vi "UDP - Write CMD.vi"(6 "V2":bool, 7 "CMD":T6, 8 "error in":errorcluster, 10 "Data":T5={"Test"={"Target Load"=0.0, "Target Disp"=0.0, "Rate"=0.0, "Speed"=0.0}, "Sensor"={"Name"=[], "Unit"=[], "Decimal Point"=[], "Ch Log"=[], "H Alarm"=[], "L Alarm"=[], "H Limit"=[], "L Limit"=[], "Filter"=[], "Gain"=[], "Calib Type"=[]}, "PID"={"SP"=-2.7823365e-08, "PV"=-3.023652e-13, "kP"=8.5432666e-24, "kI"=2.29252e-41, "kD"=1.570387e-38, "FF"=25.0, "Err Band"=0.0, "Max"=15, "Min"=-7, "Ts"=1886611780, "Out"=0, "Mode"=0}, "ADC"={"Active Ch"=[255, 255, 255, 0, 0, 0, 0, 0], "Filter Type"=2, "Post Filter"=[1, 1, 1, 1, 0, 200, 66, 184], "Gain"=[0, 0, 0, 0, 0, 122, 68, 0], "FS"=32, "IntOC"=0, "IntFC"=255, "SysOC"=255, "Cofficient"=[1.0, 1.0, 1.0, 1.0, 1.0, 1.0, 1.0, 1.0], "K"=[1.2450000047683716, 1.2450000047683716], "Max"=1048576}, "System"={"Out Type"=0, "Inverse"=0, "Monitor"=0, "Reserve"=0, "ACC Time"=0, "Pulse Rev"=0, "Stroke"=0, "Auto Off"=0, "Gear Ratio"=0.0, "Pitch"=0.0, "Max Speed"=0, "Jog Speed"=0, "Disp Coff"=0.0, "Max Load"=0}, "Index"=enum."Ch1", "Datalog"=enum."Empty"}, 11 "UDP Info":T7) -> (0 "error out":errorcluster, 1 "IP Address":string, 2 "Data Out":T4 {"Status" items=["Stop", "Ramp Up", "Ramp Down", "Jog Up", "Jog Down", "PID Mode", "PID Ramp"]; "Event" items=["Stop", "Running", "PID", "Up Limit", "Down Limit", "Load Limit"]}, 3 "UDP Info Out":T7, 4 "Success":bool, 5 "data out":string, 9 "Channels 2":T1)   [LabVIEW 2019]
uses:
  Controls/UDP - Command.ctl
  Controls/Communication - Write Data.ctl
  Controls/UDP - Status.ctl
  Controls/UDP - Event.ctl
  Controls/Global - Data UDP.vi
panel:
  out "x+y":i32
  out "appended array":u8[](array[numeric])
  out "CMD":string
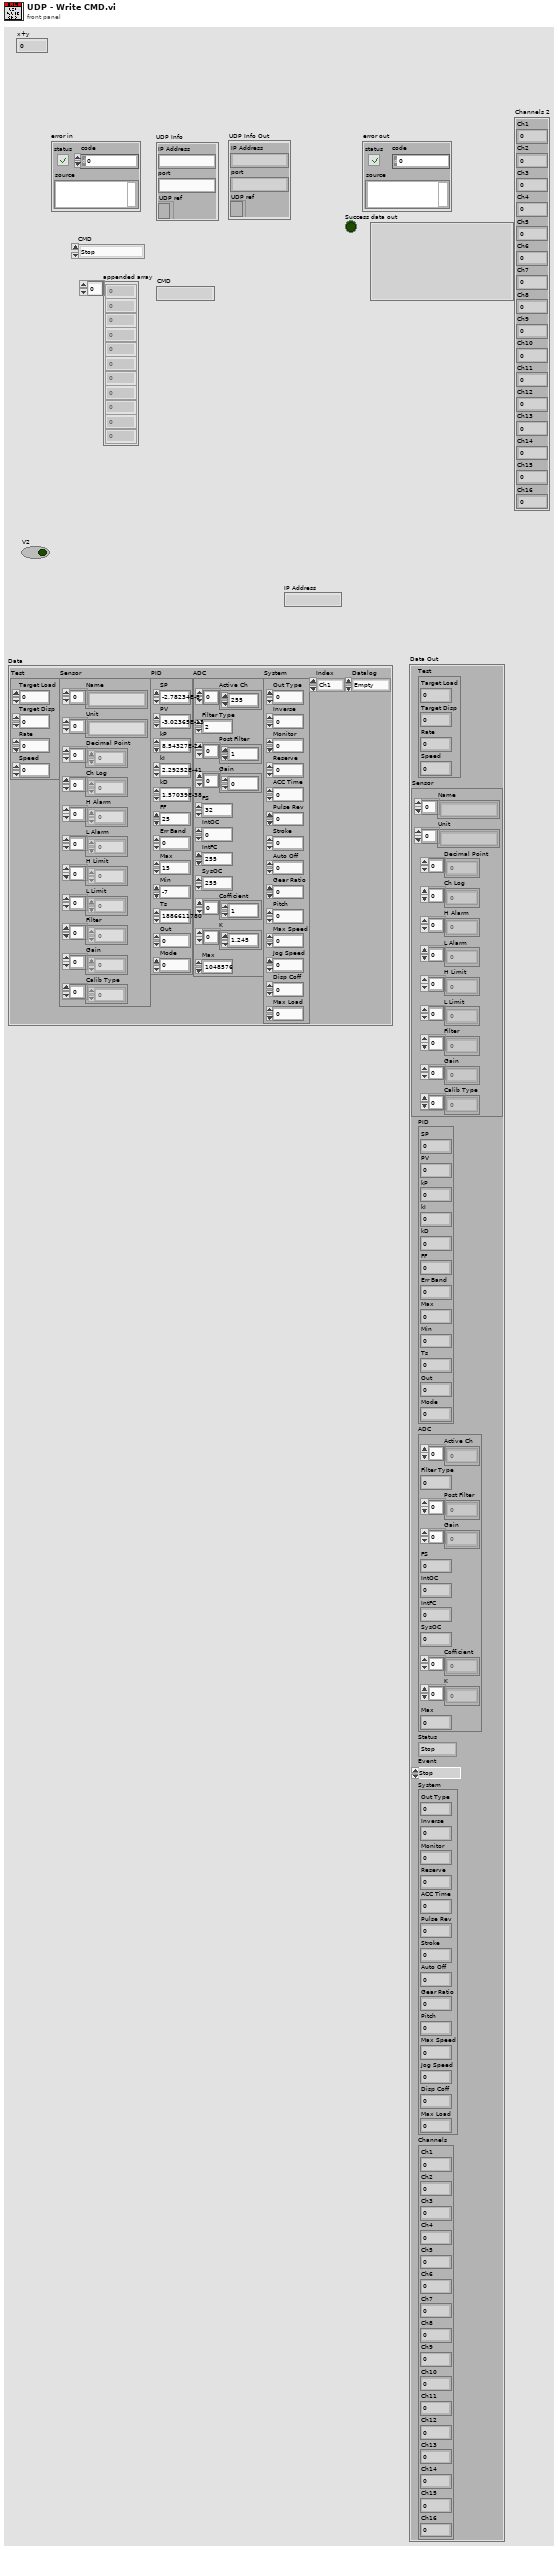
[diagram p1: front panel]
types:
  T1 = cluster{"Ch1":sgl, "Ch2":sgl, "Ch3":sgl, "Ch4":sgl, "Ch5":sgl, "Ch6":sgl, "Ch7":sgl, "Ch8":sgl, "Ch9":sgl, "Ch10":sgl, "Ch11":sgl, "Ch12":sgl, "Ch13":sgl, "Ch14":sgl, "Ch15":sgl, "Ch16":sgl}
  T2 = typedef "UDP - Status.ctl" = u16
  T3 = typedef "UDP - Event.ctl" = u16
  T4 = cluster{"Test":cluster{"Target Load":sgl, "Target Disp":sgl, "Rate":sgl, "Speed":sgl}, "Sensor":cluster{"Name":string[], "Unit":string[], "Decimal Point":u8[], "Ch Log":u8[], "H Alarm":u8[], "L Alarm":u8[], "H Limit":sgl[], "L Limit":sgl[], "Filter":u8[], "Gain":u8[], "Calib Type":u32[]}, "PID":cluster{"SP":sgl, "PV":sgl, "kP":sgl, "kI":sgl, "kD":sgl, "FF":sgl, "Err Band":sgl, "Max":i32, "Min":i32, "Ts":u32, "Out":i32, "Mode":u8}, "ADC":cluster{"Active Ch":u8[], "Filter Type":u8, "Post Filter":u8[], "Gain":u8[], "FS":u16, "IntOC":u8, "IntFC":u8, "SysOC":u8, "Cofficient":dbl[], "K":dbl[], "Max":i32}, "Status":T2, "Event":T3, "System":cluster{"Out Type":u8, "Inverse":u8, "Monitor":u8, "Reserve":u8, "ACC Time":u32, "Pulse Rev":u32, "Stroke":u32, "Auto Off":u32, "Gear Ratio":sgl, "Pitch":sgl, "Max Speed":u32, "Jog Speed":u32, "Disp Coff":sgl, "Max Load":u32}, "Channels":cluster{"Ch1":sgl, "Ch2":sgl, "Ch3":sgl, "Ch4":sgl, "Ch5":sgl, "Ch6":sgl, "Ch7":sgl, "Ch8":sgl, "Ch9":sgl, "Ch10":sgl, "Ch11":sgl, "Ch12":sgl, "Ch13":sgl, "Ch14":sgl, "Ch15":sgl, "Ch16":sgl}}
  T5 = typedef "Communication - Write Data.ctl" = cluster{"Test":cluster{"Target Load":sgl, "Target Disp":sgl, "Rate":sgl, "Speed":sgl}, "Sensor":cluster{"Name":string[], "Unit":string[], "Decimal Point":u8[], "Ch Log":u8[], "H Alarm":u8[], "L Alarm":u8[], "H Limit":sgl[], "L Limit":sgl[], "Filter":u8[], "Gain":u8[], "Calib Type":u32[]}, "PID":cluster{"SP":sgl, "PV":sgl, "kP":sgl, "kI":sgl, "kD":sgl, "FF":sgl, "Err Band":sgl, "Max":i32, "Min":i32, "Ts":u32, "Out":i32, "Mode":u8}, "ADC":cluster{"Active Ch":u8[], "Filter Type":u8, "Post Filter":u8[], "Gain":u8[], "FS":u16, "IntOC":u8, "IntFC":u8, "SysOC":u8, "Cofficient":dbl[], "K":dbl[], "Max":i32}, "System":cluster{"Out Type":u8, "Inverse":u8, "Monitor":u8, "Reserve":u8, "ACC Time":u32, "Pulse Rev":u32, "Stroke":u32, "Auto Off":u32, "Gear Ratio":sgl, "Pitch":sgl, "Max Speed":u32, "Jog Speed":u32, "Disp Coff":sgl, "Max Load":u32}, "Index":enum16{"Ch1", "Ch2", "Ch3", "Ch4", "Ch5", "Ch6", "Ch7", "Ch8", "Ch9", "Ch10", "Ch11", "Ch12", "Ch13", "Ch14", "Ch15", "Ch16"}, "Datalog":enum16{"Ch1-Ch16", "Ch17-Ch32", "Ch32-Ch48", "Ch49-Ch64", "Empty"}}
  T6 = typedef "UDP - Command.ctl" = enum16{"Stop", "Jog Up", "Jog Down", "Ramp Up", "Ramp Down", "PID Target", "PID Ramp", "Disp Run", "Read Ch Data", "Zero Channel", "Zero Disp", "Read Sensor", "Write Sensor", "Read ADC", "Write ADC", "Read PID", "Write PID", "Read Test", "Write Test", "Read System", "Write System", "Read Datalog", "Read Datalog Sensor"}
  T7 = cluster{"IP Address":string, "port":string, "UDP ref":refnum<k16>}
  T8 = cluster{"Out Type":u8, "Inverse":u8, "Monitor":u8, "Reserve":u8, "ACC Time":u32, "Pulse Rev":u32, "Stroke":u32, "Auto Off":u32, "Gear Ratio":sgl, "Pitch":sgl, "Max Speed":u32, "Jog Speed":u32, "Disp Coff":sgl, "Max Load":u32}
  T9 = cluster{"Name":string[], "Unit":string[], "Decimal Point":u8[], "Ch Log":u8[], "H Alarm":u8[], "L Alarm":u8[], "H Limit":sgl[], "L Limit":sgl[], "Filter":u8[], "Gain":u8[], "Calib Type":u32[]}
  T10 = cluster{"Active Ch":u8[], "Filter Type":u8, "Post Filter":u8[], "Gain":u8[], "FS":u16, "IntOC":u8, "IntFC":u8, "SysOC":u8, "Cofficient":dbl[], "K":dbl[], "Max":i32}
  T11 = cluster{"Target Load":sgl, "Target Disp":sgl, "Rate":sgl, "Speed":sgl}
  T12 = cluster{"SP":sgl, "PV":sgl, "kP":sgl, "kI":sgl, "kD":sgl, "FF":sgl, "Err Band":sgl, "Max":i32, "Min":i32, "Ts":u32, "Out":i32, "Mode":u8}
  T13 = cluster{"Target Load":sgl, "Target Disp":sgl, "Rate":sgl, "Ch4":sgl}
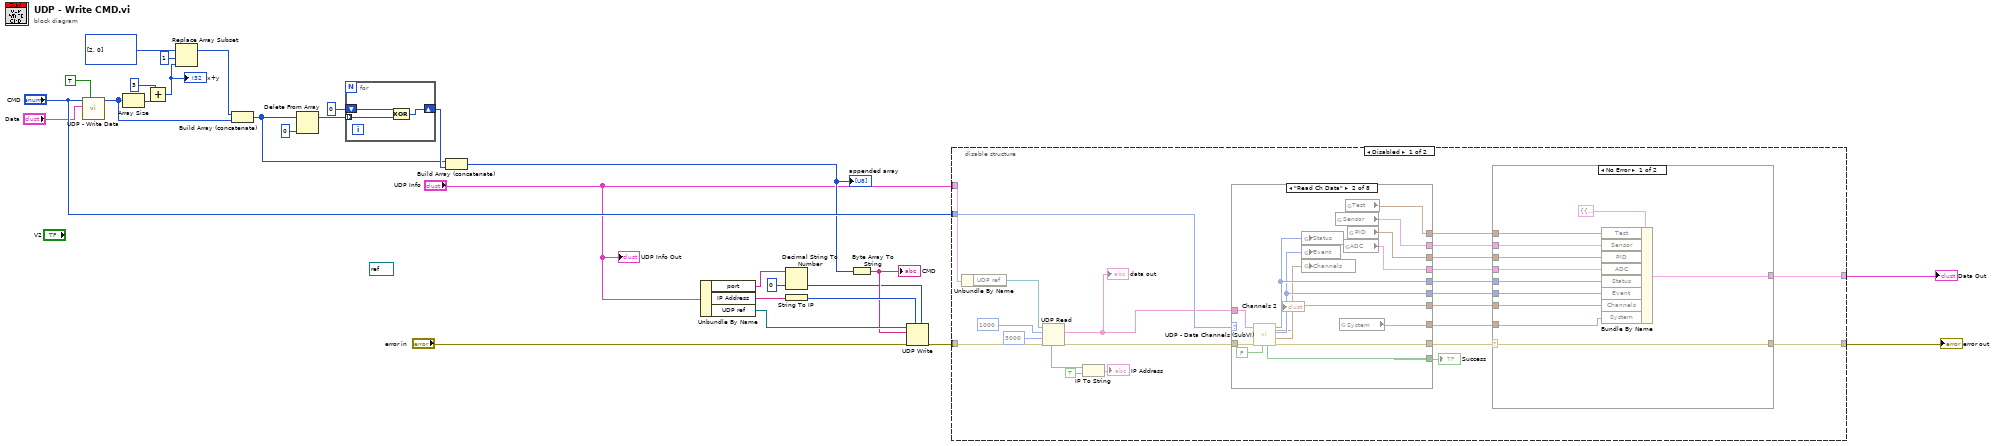
[diagram p0: block diagram]
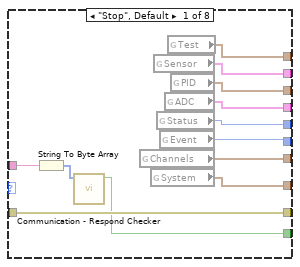
[diagram p2: hidden frame]
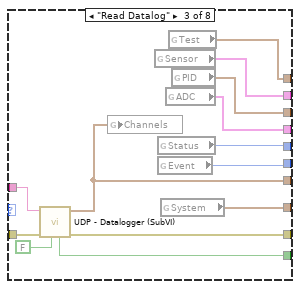
[diagram p3: hidden frame]
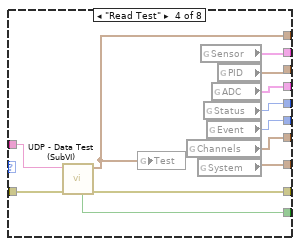
[diagram p4: hidden frame]
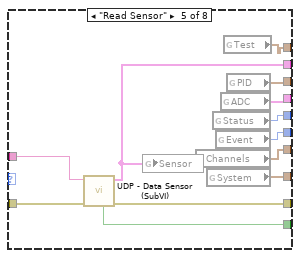
[diagram p5: hidden frame]
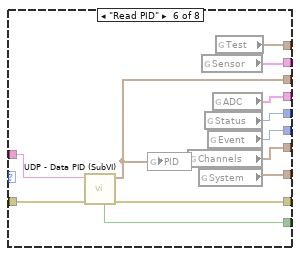
[diagram p6: hidden frame]
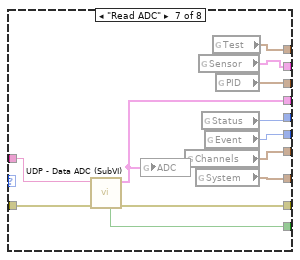
[diagram p7: hidden frame]
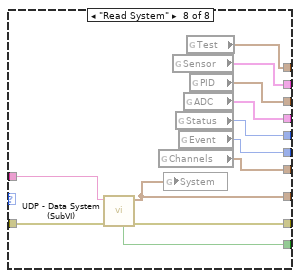
[diagram p8: hidden frame]
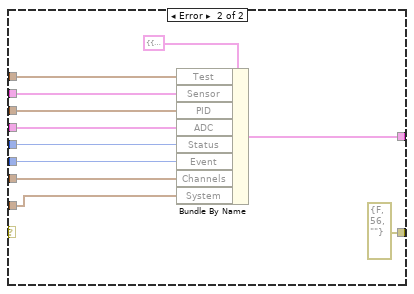
[diagram p9: hidden frame]
diagram:
  (unwired) refnum<visa-resource-name> refnum ("VISA Ref")
  n1 = call "UDP - Write Data.vi"("V2"=TRUE, "Data"="Data", "CMD"="CMD") -> ("Array"=w27:u8[])  [unwired: 8 in]
  n2 = Array Size(array=w27) -> (size(s)=w15:i32)
  n3 = Add(x=3, y=w15) -> (x+y=w13:i32)
  "x+y" <- w13
  n4 = Replace Array Subset(array=u8[] [2, 0], new element=w13, index=1) -> (w16:u8[])
  n5 = Build Array (concatenate)(w16, w27) -> (w12:u8[])
  n6 = Delete From Array(array=w12, index=0) -> (array with subset deleted=w21:u8[])  [unwired: 1 in, 1 out]
  n7 = for {
    shift-right: [w30] -> w20
    shift-left: u8 0 ("Numeric") -> [w31]
    tunnel: w21 -> [w29] mode=indexing
    n8 = Exclusive Or(1:w29, 2:w31) -> (0:w30:u8)
  }
  n9 = Build Array (concatenate)(w12, w20) -> (w19:u8[])
  "appended array" <- w19
  n10 = Unbundle By Name("UDP Info") -> ("port"=w4:string, "IP Address"=w7:string, "UDP ref"=w8:refnum<k16>)
  n11 = Decimal String To Number(string=w4, default (0L)=u16 0 ("port or service name")) -> (number=w2:u16)  [unwired: 1 in, 1 out]
  n12 = String To IP(1:w7) -> (0:w6:u32)
  n13 = Byte Array To String(unsigned byte array=w19) -> (string=w5:string)
  "CMD" <- w5
  n14 = UDP Write(address=w6, port or service name=w2, connection ID=w8, data in=w5, 8:"error in") -> (error out=w9:errorcluster)  [unwired: 1 in, 1 out]
  n15 = disable-structure shown="Disabled" {
    disable-tunnel: [w54 w176] -> w28
    disable-tunnel: "CMD" -> [w53 _]
    disable-tunnel: [w52 _] -> w24
    disable-tunnel: "UDP Info" -> [w51 _]
    disable-tunnel: w9 -> [w50 w176]
    frame Disabled {
      n16 = Unbundle By Name(w51) -> ("UDP ref"=w36:refnum<k16>)
      n17 = UDP Read(connection ID=w36, max size (548)=1000, timeout ms (25000)=3000, 8:w50) -> (data out=w38:string, error out=w49:errorcluster, 6:w35:u32)  [unwired: 2 out]
      "data out" <- w38
      n18 = IP To String(1:TRUE ("dot notation? (F)"), 2:w35) -> (0:→"IP Address":string)
      n19 = case shown="\"Read Ch Data\"" w53 {
        tunnel: w38 -> [w65 w80 w93 w105 w115 w127 w139 w151]
        tunnel: w49 -> [w66 w79 w92 w104 w117 w129 w141 w153]
        tunnel: [w66 w78 w91 w103 w116 w128 w140 w152] -> w48
        tunnel: [w63 w77 w90 w102 w114 w126 w138 w150] -> w47
        tunnel: [w60 w76 w82 w99 w109 w121 w133 w146] -> w46
        tunnel: [w61 w75 w81 w100 w108 w120 w132 w147] -> w45
        tunnel: [w62 w74 w83 w95 w107 w119 w131 w148] -> w44
        tunnel: [w56 w70 w86 w101 w112 w123 w135 w142] -> w43
        tunnel: [w57 w71 w87 w96 w113 w124 w134 w143] -> w42
        tunnel: [w58 w72 w88 w97 w111 w125 w136 w144] -> w41
        tunnel: [w59 w73 w89 w98 w110 w122 w137 w145] -> w40
        tunnel: [w55 w69 w85 w94 w106 w118 w130 w149] -> w39
        frame "Stop", Default {
          n20 = String To Byte Array(string=w65) -> (unsigned byte array=w64:u8[])
          n21 = call "Communication - Respond Checker.vi"("Read Data"=w64) -> ("Success"=w63:bool)  [unwired: 10 in]
          n22 = global read "Global - Data UDP.vi" "Channels"() -> (w62:T1)
          n23 = global read "Global - Data UDP.vi" "System"() -> (w55:T8)
          n24 = global read "Global - Data UDP.vi" "Sensor"() -> (w57:T9)
          n25 = global read "Global - Data UDP.vi" "Status"() -> (w60:T2)
          n26 = global read "Global - Data UDP.vi" "Event"() -> (w61:T3)
          n27 = global read "Global - Data UDP.vi" "ADC"() -> (w59:T10)
          n28 = global read "Global - Data UDP.vi" "Test"() -> (w56:T11)
          n29 = global read "Global - Data UDP.vi" "PID"() -> (w58:T12)
        }
        frame "Read Ch Data" {
          n30 = call "UDP - Data Channels (SubVI).vi"("test?"=FALSE, "error in"=w79, "data in"=w80) -> ("error out"=w78:errorcluster, "Channels"=w74:T1, "Event"=w75:T3, "Status"=w76:T2, "Success"=w77:bool, "Channels 2"=→"Channels 2":T1)  [unwired: 3 in]
          n31 = global write "Global - Data UDP.vi" "Status"(w76) -> ()
          n32 = global write "Global - Data UDP.vi" "Event"(w75) -> ()
          n33 = global write "Global - Data UDP.vi" "Channels"(w74) -> ()
          n34 = global read "Global - Data UDP.vi" "Sensor"() -> (w71:T9)
          n35 = global read "Global - Data UDP.vi" "System"() -> (w69:T8)
          n36 = global read "Global - Data UDP.vi" "ADC"() -> (w73:T10)
          n37 = global read "Global - Data UDP.vi" "Test"() -> (w70:T11)
          n38 = global read "Global - Data UDP.vi" "PID"() -> (w72:T12)
        }
        frame "Read Datalog" {
          n39 = call "UDP - Datalogger (SubVI).vi"("test?"=FALSE, "error in"=w92, "data in"=w93) -> ("error out"=w91:errorcluster, "Channels"=w83:T1, "Success"=w90:bool)  [unwired: 6 in]
          n40 = global write "Global - Data UDP.vi" "Channels"(w83) -> ()
          n41 = global read "Global - Data UDP.vi" "Sensor"() -> (w87:T9)
          n42 = global read "Global - Data UDP.vi" "Status"() -> (w82:T2)
          n43 = global read "Global - Data UDP.vi" "Event"() -> (w81:T3)
          n44 = global read "Global - Data UDP.vi" "System"() -> (w85:T8)
          n45 = global read "Global - Data UDP.vi" "ADC"() -> (w89:T10)
          n46 = global read "Global - Data UDP.vi" "Test"() -> (w86:T11)
          n47 = global read "Global - Data UDP.vi" "PID"() -> (w88:T12)
        }
        frame "Read Test" {
          n48 = call "UDP - Data Test (SubVI).vi"("error in"=w104, "data in"=w105) -> ("error out"=w103:errorcluster, "Data Test"=w101:T13, "Success"=w102:bool)  [unwired: 7 in]
          n49 = global write "Global - Data UDP.vi" "Test"(w101) -> ()
          n50 = global read "Global - Data UDP.vi" "Channels"() -> (w95:T1)
          n51 = global read "Global - Data UDP.vi" "System"() -> (w94:T8)
          n52 = global read "Global - Data UDP.vi" "Sensor"() -> (w96:T9)
          n53 = global read "Global - Data UDP.vi" "Status"() -> (w99:T2)
          n54 = global read "Global - Data UDP.vi" "Event"() -> (w100:T3)
          n55 = global read "Global - Data UDP.vi" "ADC"() -> (w98:T10)
          n56 = global read "Global - Data UDP.vi" "PID"() -> (w97:T12)
        }
        frame "Read Sensor" {
          n57 = call "UDP - Data Sensor (SubVI).vi"("error in"=w117, "String"=w115) -> ("error out"=w116:errorcluster, "Sensor Out"=w113:T9, "Success"=w114:bool)  [unwired: 7 in]
          n58 = global write "Global - Data UDP.vi" "Sensor"(w113) -> ()
          n59 = global read "Global - Data UDP.vi" "Channels"() -> (w107:T1)
          n60 = global read "Global - Data UDP.vi" "System"() -> (w106:T8)
          n61 = global read "Global - Data UDP.vi" "Status"() -> (w109:T2)
          n62 = global read "Global - Data UDP.vi" "Event"() -> (w108:T3)
          n63 = global read "Global - Data UDP.vi" "ADC"() -> (w110:T10)
          n64 = global read "Global - Data UDP.vi" "Test"() -> (w112:T11)
          n65 = global read "Global - Data UDP.vi" "PID"() -> (w111:T12)
        }
        frame "Read PID" {
          n66 = call "UDP - Data PID (SubVI).vi"("error in (no error)"=w129, "Data"=w127) -> ("error out"=w128:errorcluster, "PID Setting"=w125:T12, "Success"=w126:bool)  [unwired: 7 in]
          n67 = global write "Global - Data UDP.vi" "PID"(w125) -> ()
          n68 = global read "Global - Data UDP.vi" "Channels"() -> (w119:T1)
          n69 = global read "Global - Data UDP.vi" "System"() -> (w118:T8)
          n70 = global read "Global - Data UDP.vi" "Sensor"() -> (w124:T9)
          n71 = global read "Global - Data UDP.vi" "Status"() -> (w121:T2)
          n72 = global read "Global - Data UDP.vi" "Event"() -> (w120:T3)
          n73 = global read "Global - Data UDP.vi" "ADC"() -> (w122:T10)
          n74 = global read "Global - Data UDP.vi" "Test"() -> (w123:T11)
        }
        frame "Read ADC" {
          n75 = call "UDP - Data ADC (SubVI).vi"("error in (no error)"=w141, "Data"=w139) -> ("error out"=w140:errorcluster, "Data ADC"=w137:T10, "Success"=w138:bool)  [unwired: 7 in]
          n76 = global write "Global - Data UDP.vi" "ADC"(w137) -> ()
          n77 = global read "Global - Data UDP.vi" "Channels"() -> (w131:T1)
          n78 = global read "Global - Data UDP.vi" "System"() -> (w130:T8)
          n79 = global read "Global - Data UDP.vi" "Sensor"() -> (w134:T9)
          n80 = global read "Global - Data UDP.vi" "Status"() -> (w133:T2)
          n81 = global read "Global - Data UDP.vi" "Event"() -> (w132:T3)
          n82 = global read "Global - Data UDP.vi" "Test"() -> (w135:T11)
          n83 = global read "Global - Data UDP.vi" "PID"() -> (w136:T12)
        }
        frame "Read System" {
          n84 = call "UDP - Data System (SubVI).vi"("error in (no error)"=w153, "Data"=w151) -> ("error out"=w152:errorcluster, "Data System"=w149:T8, "Success"=w150:bool)  [unwired: 7 in]
          n85 = global read "Global - Data UDP.vi" "Channels"() -> (w148:T1)
          n86 = global write "Global - Data UDP.vi" "System"(w149) -> ()
          n87 = global read "Global - Data UDP.vi" "Sensor"() -> (w143:T9)
          n88 = global read "Global - Data UDP.vi" "Status"() -> (w146:T2)
          n89 = global read "Global - Data UDP.vi" "Event"() -> (w147:T3)
          n90 = global read "Global - Data UDP.vi" "ADC"() -> (w145:T10)
          n91 = global read "Global - Data UDP.vi" "Test"() -> (w142:T11)
          n92 = global read "Global - Data UDP.vi" "PID"() -> (w144:T12)
        }
      }
      "Success" <- w47
      n93 = case shown="No Error" w48 {
        selector: w48 -> [w164 _]
        tunnel: [w164 errorcluster {"status"=FALSE, "code"=56, "source"=""} ("error IO")] -> w54
        tunnel: w46 -> [w162 w169]
        tunnel: w45 -> [w161 w168]
        tunnel: w44 -> [w160 w167]
        tunnel: w43 -> [w159 w173]
        tunnel: w42 -> [w158 w172]
        tunnel: w41 -> [w157 w171]
        tunnel: w40 -> [w156 w170]
        tunnel: w39 -> [w155 w166]
        tunnel: [w154 w165] -> w52
        frame No Error {
          n94 = Bundle By Name(cluster=T4 {"Test"={"Target Load"=0.0, "Target Disp"=0.0, "Rate"=0.0, "Speed"=0.0}, "Sensor"={"Name"=[], "Unit"=[], "Decimal Point"=[], "Ch Log"=[], "H Alarm"=[], "L Alarm"=[], "H Limit"=[], "L Limit"=[], "Filter"=[], "Gain"=[], "Calib Type"=[]}, "PID"={"SP"=-2.7823365e-08, "PV"=-3.023652e-13, "kP"=8.5432666e-24, "kI"=2.29252e-41, "kD"=1.570387e-38, "FF"=25.0, "Err Band"=0.0, "Max"=15, "Min"=-7, "Ts"=1886611780, "Out"=0, "Mode"=0}, "ADC"={"Active Ch"=[255, 255, 255, 0, 0, 0, 0, 0], "Filter Type"=2, "Post Filter"=[1, 1, 1, 1, 0, 200, 66, 184], "Gain"=[0, 0, 0, 0, 0, 122, 68, 0], "FS"=32, "IntOC"=0, "IntFC"=255, "SysOC"=255, "Cofficient"=[1.0, 1.0, 1.0, 1.0, 1.0, 1.0, 1.0, 1.0], "K"=[1.2450000047683716, 1.2450000047683716], "Max"=1048576}, "Status"=0, "Event"=0, "System"={"Out Type"=0, "Inverse"=0, "Monitor"=0, "Reserve"=0, "ACC Time"=0, "Pulse Rev"=0, "Stroke"=0, "Auto Off"=0, "Gear Ratio"=0.0, "Pitch"=0.0, "Max Speed"=0, "Jog Speed"=0, "Disp Coff"=0.0, "Max Load"=0}, "Channels"={"Ch1"=0.0, "Ch2"=0.0, "Ch3"=0.0, "Ch4"=0.0, "Ch5"=0.0, "Ch6"=0.0, "Ch7"=0.0, "Ch8"=0.0, "Ch9"=0.0, "Ch10"=0.0, "Ch11"=0.0, "Ch12"=0.0, "Ch13"=0.0, "Ch14"=0.0, "Ch15"=0.0, "Ch16"=0.0}} ("Data out"), "Test"=w159, "Sensor"=w158, "PID"=w157, "ADC"=w156, "Status"=w162, "Event"=w161, "Channels"=w160, "System"=w155) -> (w154:T4)
        }
        frame Error {
          n95 = Bundle By Name(cluster=T4 {"Test"={"Target Load"=0.0, "Target Disp"=0.0, "Rate"=0.0, "Speed"=0.0}, "Sensor"={"Name"=[], "Unit"=[], "Decimal Point"=[], "Ch Log"=[], "H Alarm"=[], "L Alarm"=[], "H Limit"=[], "L Limit"=[], "Filter"=[], "Gain"=[], "Calib Type"=[]}, "PID"={"SP"=-2.7823365e-08, "PV"=-3.023652e-13, "kP"=8.5432666e-24, "kI"=2.29252e-41, "kD"=1.570387e-38, "FF"=25.0, "Err Band"=0.0, "Max"=15, "Min"=-7, "Ts"=1886611780, "Out"=0, "Mode"=0}, "ADC"={"Active Ch"=[255, 255, 255, 0, 0, 0, 0, 0], "Filter Type"=2, "Post Filter"=[1, 1, 1, 1, 0, 200, 66, 184], "Gain"=[0, 0, 0, 0, 0, 122, 68, 0], "FS"=32, "IntOC"=0, "IntFC"=255, "SysOC"=255, "Cofficient"=[1.0, 1.0, 1.0, 1.0, 1.0, 1.0, 1.0, 1.0], "K"=[1.2450000047683716, 1.2450000047683716], "Max"=1048576}, "Status"=0, "Event"=0, "System"={"Out Type"=0, "Inverse"=0, "Monitor"=0, "Reserve"=0, "ACC Time"=0, "Pulse Rev"=0, "Stroke"=0, "Auto Off"=0, "Gear Ratio"=0.0, "Pitch"=0.0, "Max Speed"=0, "Jog Speed"=0, "Disp Coff"=0.0, "Max Load"=0}, "Channels"={"Ch1"=0.0, "Ch2"=0.0, "Ch3"=0.0, "Ch4"=0.0, "Ch5"=0.0, "Ch6"=0.0, "Ch7"=0.0, "Ch8"=0.0, "Ch9"=0.0, "Ch10"=0.0, "Ch11"=0.0, "Ch12"=0.0, "Ch13"=0.0, "Ch14"=0.0, "Ch15"=0.0, "Ch16"=0.0}} ("Data out"), "Test"=w173, "Sensor"=w172, "PID"=w171, "ADC"=w170, "Status"=w169, "Event"=w168, "Channels"=w167, "System"=w166) -> (w165:T4)
        }
      }
    }
    frame Enabled {
    }
  }
  "error out" <- w28
  "Data Out" <- w24
  "UDP Info Out" <- "UDP Info"
